vi "Append New Paragraph.vi"(8 "error in (no error)":errorcluster, 9 "Paragraph.Style":refnum<class "Style.lvclass">, 10 "Paragraph.Text":string, 11 "xwpfDocument in":refnum<class "xwpfDocument.lvclass">) -> (0 "error out":errorcluster, 3 "xwpfDocument out":refnum<class "xwpfDocument.lvclass">)   [LabVIEW 2017, in "Word_Specific.lvlib" / "xwpfDocument.lvclass"]
uses:
  xwpfDocument.lvclass
  Styles/Style/Style.lvclass
  xwpfDocument.lvclass/xwpfDocument.ctl
  C:/Users/Neo/Desktop/Dev_Tools_BR/LabVIEW_NPOI/lib/NPOI 2.1.1/NPOI.OOXML.dll
  lib/NPOI 2.1.1/NPOI.OOXML.dll
  xwpfParagraph/xwpfParagraph.lvclass
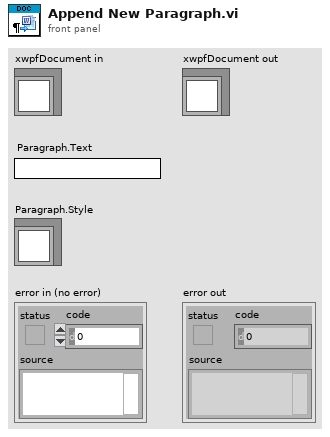
[diagram p1: front panel]
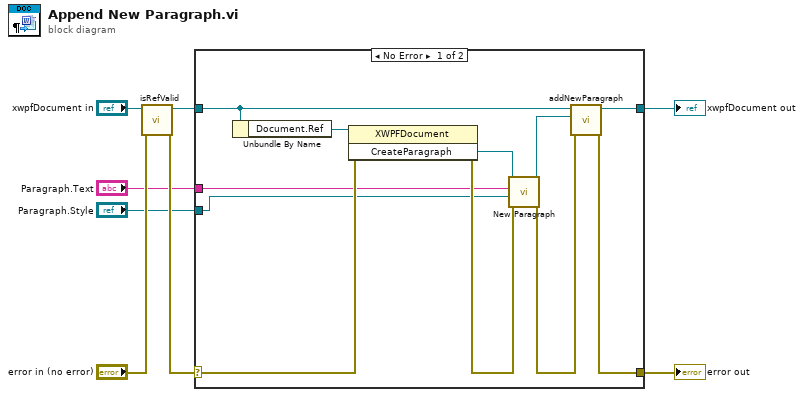
[diagram p0: block diagram]
diagram:
  n1 = call-dynamic "isRefValid.vi"("error in (no error)"="error in (no error)", "xwpfDocument in"="xwpfDocument in") -> ("error out"=w3:errorcluster, "xwpfDocument out"=w5:refnum<class "xwpfDocument.lvclass">)  [unwired: 8 in]
  n2 = case shown="No Error" w3 {
    selector: w3 -> [w17 w21]
    tunnel: [w11 w21] -> w8
    tunnel: [w14 w20] -> w6
    tunnel: w5 -> [w15 w20]
    tunnel: "Paragraph.Text" -> [w10 _]
    tunnel: "Paragraph.Style" -> [w9 _]
    frame No Error {
      n3 = Unbundle By Name(w15) -> ("Document.Ref"=w19:refnum<k24>)
      n4 = invoke class="XWPFDocument" method="CreateParagraph"(reference=w19, error in=w17) -> (error out=w16:errorcluster, "CreateParagraph"=w18:refnum<k24>)  [unwired: 1 in, 1 out]
      n5 = call "New Paragraph.vi"("error in (no error)"=w16, "Paragraph.Style"=w9, "Paragraph.Text"=w10, "Paragraph.Ref"=w18) -> ("error out"=w12:errorcluster, "xwpfParagraph out"=w13:refnum<class "xwpfParagraph.lvclass">)  [unwired: 6 in]
      n6 = call "addNewParagraph.vi"("error in (no error)"=w12, "New Paragraph"=w13, "xwpfDocument in"=w15) -> ("error out"=w11:errorcluster, "xwpfDocument out"=w14:refnum<class "xwpfDocument.lvclass">)  [unwired: 7 in]
    }
    frame Error {
    }
  }
  "error out" <- w8
  "xwpfDocument out" <- w6
